vi "Get Color Array.vi"(7 "Alpha":sgl, 9 "Color Index Array":i32[](array[numeric]), 11 "Color Ramp Cluster":T1={"Color Ramp Style"=enum."None", "Color Ramp Array"=[16711934, 393471, 57855, 4390754, 16449346, 16744722, 16711680], "Color Ramp Index"=[45, 91, 133, 175, 219, 255], "Interpolate?"=FALSE, "Logarithm?"=FALSE}) -> (1 "Color Binding Mode":T2(ring), 3 "Color Array":cluster{"R":sgl, "G":sgl, "B":sgl, "A":sgl}[](array[cluster]))   [LabVIEW 2020, in "3D Plot.lvclass"]
uses:
  3D Plot.lvclass
  Color Ramp Cluster.ctl
  NI_3D Picture Control.lvlib
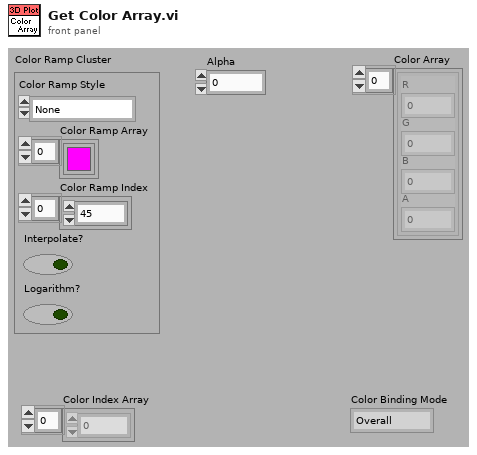
[diagram p1: front panel]
types:
  T1 = typedef "3D Plot.lvclass/Color Ramp Cluster.ctl" = cluster{"Color Ramp Style":enum16{"None", "Shaded", "Color spectrum", "Grey scale", "Custom"}, "Color Ramp Array":u32[], "Color Ramp Index":i32[], "Interpolate?":bool, "Logarithm?":bool}
  T2 = enum16{"Overall", "Per Primitive", "Per Vertex", "Binding Off"}
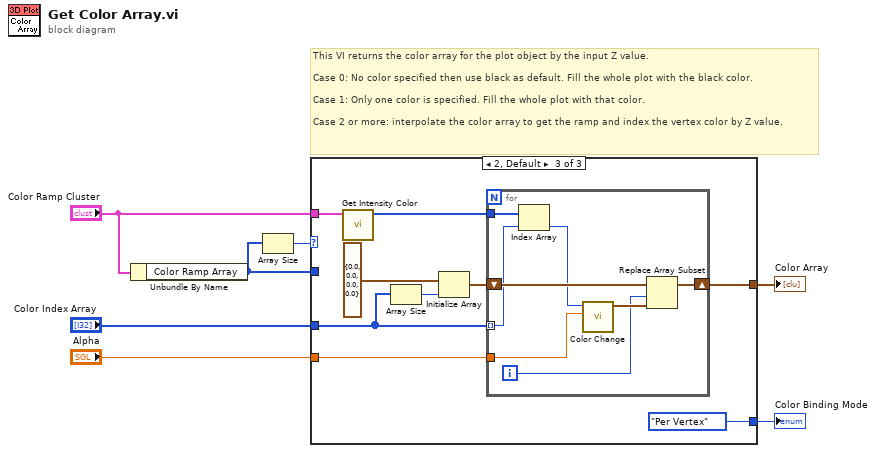
[diagram p0: block diagram]
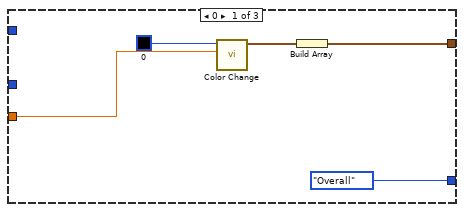
[diagram p2: hidden frame]
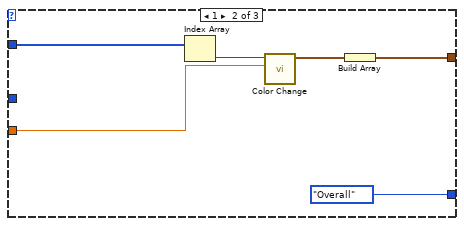
[diagram p3: hidden frame]
diagram:
  # "This VI returns the color array for the plot object by the input Z value.\n\nCase 0: No color specified then use black as default. Fill the whole plot with the black color.\n\nCase 1: Only one color is specified. Fill the whole plot with that color.\n\nCase 2 or more: interpolate the color array to get the ramp and index the vertex color by Z value."
  n1 = Unbundle By Name("Color Ramp Cluster") -> ("Color Ramp Array"=w2:u32[])
  n2 = Array Size(array=w2) -> (size(s)=w4:i32)
  n3 = case shown="2, Default" w4 {
    tunnel: w2 -> [_ w16 _]
    tunnel: "Color Index Array" -> [_ _ w21]
    tunnel: "Alpha" -> [w10 w13 w25]
    tunnel: [T2."Overall" ("Color Binding Mode") T2."Overall" ("Color Binding Mode") T2."Per Vertex" ("Color Binding Mode")] -> w6
    tunnel: [w9 w14 w26] -> w5
    tunnel: "Color Ramp Cluster" -> [_ _ w19]
    frame 0 {
      n4 = call "Color Change.vi"("Alpha"=w10, "Color"=u32 0) -> ("RGBA"=w11:cluster{"R":sgl, "G":sgl, "B":sgl, "A":sgl})  [unwired: 9 out]
      n5 = Build Array(w11) -> (w9:cluster{"R":sgl, "G":sgl, "B":sgl, "A":sgl}[])
    }
    frame 1 {
      n6 = Index Array(array=w16) -> (element=w15:u32)  [unwired: 1 in]
      n7 = call "Color Change.vi"("Alpha"=w13, "Color"=w15) -> ("RGBA"=w18:cluster{"R":sgl, "G":sgl, "B":sgl, "A":sgl})  [unwired: 9 out]
      n8 = Build Array(w18) -> (w14:cluster{"R":sgl, "G":sgl, "B":sgl, "A":sgl}[])
    }
    frame 2, Default {
      n9 = call "Get Intensity Color.vi"("Color Ramp Cluster"=w19) -> ("Intensity Color"=w24:u32[])  [unwired: 3 in, 7 out]
      n10 = Array Size(array=w21) -> (size(s)=w20:i32)
      n11 = Initialize Array(cluster{"R":sgl, "G":sgl, "B":sgl, "A":sgl} {"R"=0.0, "G"=0.0, "B"=0.0, "A"=0.0} ("RGBA"), w20) -> (w22:cluster{"R":sgl, "G":sgl, "B":sgl, "A":sgl}[])
      n12 = for {
        tunnel: w21 -> [w32] mode=indexing
        tunnel: w24 -> [w35]
        shift-right: [w33] -> w26
        shift-left: w22 -> [w34]
        tunnel: w25 -> [w30]
        i -> [w28]
        n13 = Index Array(array=w35, index=w32) -> (element=w31:u32)
        n14 = call "Color Change.vi"("Alpha"=w30, "Color"=w31) -> ("RGBA"=w29:cluster{"R":sgl, "G":sgl, "B":sgl, "A":sgl})  [unwired: 9 out]
        n15 = Replace Array Subset(array=w34, new element=w29, index=w28) -> (w33:cluster{"R":sgl, "G":sgl, "B":sgl, "A":sgl}[])
      }
    }
  }
  "Color Binding Mode" <- w6
  "Color Array" <- w5
